vi "Calc New Setpoint1.vi"(9 "-":bool, 10 "+":bool, 11 "Digital in":refnum<vi>) -> ()   [LabVIEW 2016]
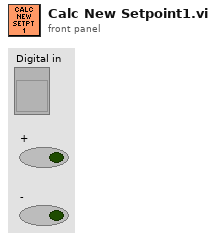
[diagram p1: front panel]
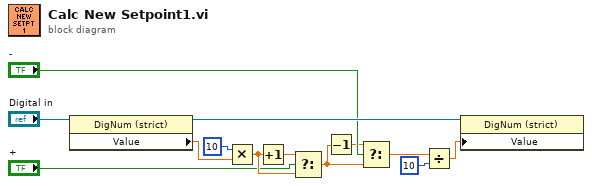
[diagram p0: block diagram]
diagram:
  n1 = property class="DigNum (strict)"(reference="Digital in") -> (reference out=w12:refnum<vi>, "Value"=w11:sgl)  [unwired: 1 in, 1 out]
  n2 = Multiply(x=10, y=w11) -> (x*y=w9:sgl)
  n3 = Increment(x=w9) -> (x+1=w2:sgl)
  n4 = Select(t=w2, s="+", f=w9) -> (s? t:f=w8:sgl)
  n5 = Decrement(x=w8) -> (x-1=w4:sgl)
  n6 = Select(t=w4, s="-", f=w8) -> (s? t:f=w7:sgl)
  n7 = Divide(x=w7, y=10) -> (x/y=w13:sgl)
  n8 = property class="DigNum (strict)"(reference=w12, "Value"=w13) -> ()  [unwired: 1 in, 2 out]
